vi "get Display Help.vi"(11 "Scene in":refnum<class "Scene.lvclass">) -> (3 "Display Help":bool)   [LabVIEW 2022 SP3, in "Application.lvlib" / "Scene.lvclass"]
uses:
  Scene.lvclass
  Scene.lvclass/Scene.ctl
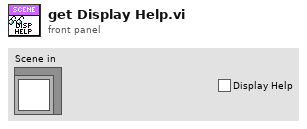
[diagram p1: front panel]
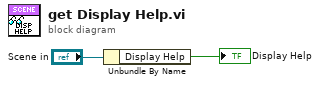
[diagram p0: block diagram]
diagram:
  n1 = Unbundle By Name("Scene in") -> ("Display Help"=→"Display Help":bool)
